vi "CVT2ReferenceWriteTest.vi"() -> (3 "Unit Test Framework Results":T1)   [LabVIEW 2013, in "UnitTests.lvlib"]
uses:
  UnitTests.lvlib
  <vilib>/utf/common/utf_test_result_troll.ctl
  <vilib>/utf/common/utf_test_result.ctl
  <vilib>/utf/common/utf_test_result_failure.ctl
  <vilib>/utf/common/utf_test_comparison_operators.ctl
  <vilib>/utf/common/utf_vi_tag.ctl
  <vilib>/NI/Current Value Table/Type Defs/Data Types.ctl
  <vilib>/NI/Current Value Table/DataTypes/I32_Write Index Set.vi
  <vilib>/NI/Current Value Table/DataTypes/I32_Read Index Set.vi
  <vilib>/NI/Current Value Table/FGVs/Tag Memory.vi
  <vilib>/NI/Current Value Table/Memory Block.vi
  <vilib>/NI/Current Value Table/DataTypes/I32_Memory Block.vi
  <vilib>/utf/NI_UnitTestFramework.lvlib
  <vilib>/NI/Current Value Table/Current Value Table.lvlib
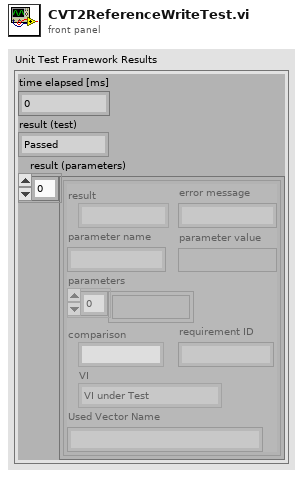
[diagram p1: front panel]
types:
  T1 = typedef "NI_UnitTestFramework.lvlib/utf_test_result_troll.ctl" = cluster{"time elapsed [ms]":u32, "result (test)":T2, "result (parameters)":T3[]}
  T2 = typedef "NI_UnitTestFramework.lvlib/utf_test_result.ctl" = enum16{"Passed", "Failed", "Error", "Skipped", "Not Processed"}
  T3 = typedef "NI_UnitTestFramework.lvlib/utf_test_result_failure.ctl" = cluster{"result":T2, "error message":string, "parameter name":string, "parameter value":variant, "parameters":variant[], "comparison":T4, "requirement ID":string, "VI":T5, "Used Vector Name":string}
  T4 = typedef "NI_UnitTestFramework.lvlib/utf_test_comparison_operators.ctl" = enum16{"=", "!=", ">", ">=", "<", "<=", "range", "symmetric tolerance", "asymmetric tolerance", "string contains", "string not contain", "array size", "string length", "array range", "by element", "array range (limit array)", "user-defined", "array contains", "array not contain", "vector length", "= (elm)", "!= (elm)", "= (case insensitive)", "!= (case insensitive)"}
  T5 = typedef "NI_UnitTestFramework.lvlib/utf_vi_tag.ctl" = enum16{"Setup VI", "VI under Test", "Teardown VI"}
  T6 = typedef "Current Value Table.lvlib/Data Types.ctl" = enum16{"Double", "Single", "I64", "I32", "I16", "I8", "U64", "U32", "U16", "U8", "String", "Boolean", "Array of U8", "Array of U16", "Array of U32", "Array of U64", "Array of I64", "Array of I32", "Array of I16", "Array of I8", "Array of Double", "Array of Single", "Array of Boolean", "Array of String"}
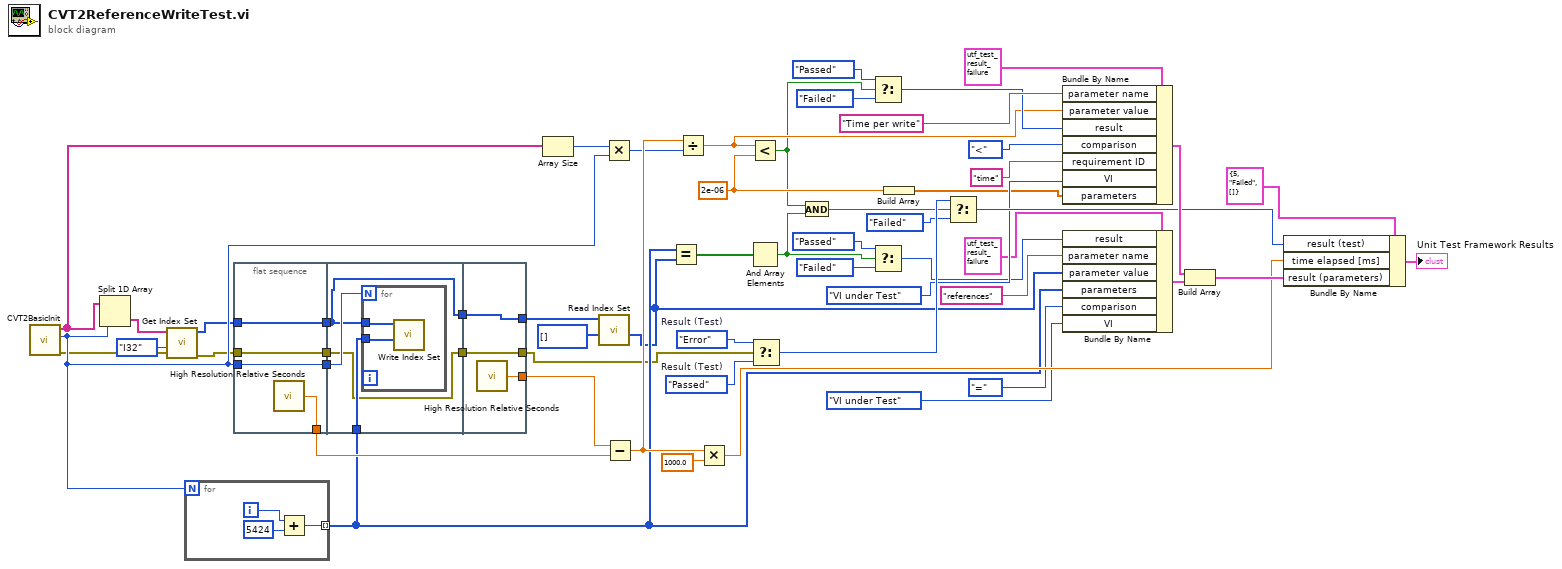
[diagram p0: block diagram]
diagram:
  w31 = 2e-06 ("y")
  w51 = utf_test_result."Error"  # Result (Test)
  w50 = utf_test_result."Passed"  # Result (Test)
  n1 = call "CVT2BasicInit.vi"() -> ("error out"=w12:errorcluster, "Tags per type out"=w13:i32, "names"=w14:string[])  [unwired: 9 in]
  n2 = Split 1D Array(array=w14, index=w13) -> (second subarray=w2:string[])  [unwired: 1 out]
  n3 = call <vilib>:"Get Index Set.vi"("error in (no error)"=w12, "Expected Type"=Data_Types."I32", "Tag Names"=w2) -> ("error out"=w11:errorcluster, "Tag References"=w9:i32[])  [unwired: 7 in]
  n4 = for {
    N: w13 -> [_]
    tunnel: [w57] -> w15 mode=indexing
    i -> [w59]
    n5 = Add(x=w59, y=5424) -> (x+y=w57:i32)
  }
  n6 = flat-sequence {
    tunnel: [w63] -> w53
    tunnel: w11 -> [w61]
    tunnel: [w62] -> w45
    tunnel: w13 -> [w62]
    tunnel: [w61] -> w44
    tunnel: w9 -> [w60]
    tunnel: [w60] -> w8
    tunnel: w45 -> [w67]
    tunnel: w44 -> [w65]
    tunnel: w15 -> [w66]
    tunnel: [w65] -> w10
    tunnel: w8 -> [w64]
    tunnel: [w64] -> w4
    tunnel: [w72] -> w54
    tunnel: [w71] -> w7
    tunnel: w10 -> [w71]
    tunnel: w4 -> [w70]
    tunnel: [w70] -> w3
    frame #0 {
      n7 = call <vilib>:"High Resolution Relative Seconds.vi"() -> ("relative seconds"=w63:dbl)
    }
    frame #1 {
      n8 = for {
        N: w67 -> [_]
        tunnel: w66 -> [w69]
        tunnel: w64 -> [w68]
        n9 = call-poly <vilib>:"Write Index Set.vi"("Values"=w69, "Indices"=w68) -> ()  [unwired: 10 in]
      }
    }
    frame #2 {
      n10 = call <vilib>:"High Resolution Relative Seconds.vi"() -> ("relative seconds"=w72:dbl)
    }
  }
  n11 = Array Size(array=w14) -> (size(s)=w26:i32)
  n12 = call-poly <vilib>:"Read Index Set.vi"("Default"=i32[] [], "Indices"=w3) -> ("Values"=w5:i32[])  [unwired: 9 in]
  n13 = Multiply(x=w26, y=w13) -> (x*y=w25:i32)
  n14 = Subtract(x=w54, y=w53) -> (x-y=w43:dbl)
  n15 = Equal?(x=w15, y=w5) -> (x = y?=w17:bool[])
  n16 = Divide(x=w43, y=w25) -> (x/y=w34:dbl)
  n17 = Multiply(x=w43, y=1000.0) -> (x*y=w46:dbl)
  n18 = Less?(x=w34, y=w31) -> (x < y?=w27:bool)
  n19 = And Array Elements(Boolean array=w17) -> (logical AND=w16:bool)
  n20 = Select(t=w51, s=w7, f=w50) -> (s? t:f=w41:T2)
  n21 = And(x=w27, y=w16) -> (x .and. y?=w28:bool)
  n22 = Select(t=utf_test_result."Passed" ("result"), s=w27, f=utf_test_result."Failed" ("result")) -> (s? t:f=w35:T2)
  n23 = Select(t=utf_test_result."Passed" ("result"), s=w16, f=utf_test_result."Failed" ("result")) -> (s? t:f=w20:T2)
  n24 = Build Array(w31) -> (w30:dbl[])
  n25 = Select(t=w41, s=w28, f=utf_test_result."Failed") -> (s? t:f=w39:T2)
  n26 = Bundle By Name(cluster=T3 {"result"=enum."Passed", "error message"="", "parameter name"="", "parameter value"=variant, "parameters"=[], "comparison"=enum."=", "requirement ID"="", "VI"=enum."Setup VI", "Used Vector Name"=""} ("Unit Test Framework - result (parameters)"), "parameter name"="Time per write", "parameter value"=w34, "result"=w35, "comparison"=utf_test_comparison_operators."<", "requirement ID"="time", "VI"=utf_vi_tag."VI under Test", "parameters"=w30) -> (w49:T3)
  n27 = Bundle By Name(cluster=T3 {"result"=enum."Passed", "error message"="", "parameter name"="", "parameter value"=variant, "parameters"=[], "comparison"=enum."=", "requirement ID"="", "VI"=enum."Setup VI", "Used Vector Name"=""} ("Unit Test Framework - result (parameters)"), "result"=w20, "parameter name"="references" ("format string"), "parameter value"=w5, "parameters"=w15, "comparison"=utf_test_comparison_operators."=", "VI"=utf_vi_tag."VI under Test") -> (w29:T3)
  n28 = Build Array(w49, w29) -> (w48:T3[])
  n29 = Bundle By Name(cluster=T1 {"time elapsed [ms]"=5, "result (test)"=enum."Failed", "result (parameters)"=[]} ("Unit Test Framework - Result"), "result (test)"=w39, "time elapsed [ms]"=w46, "result (parameters)"=w48) -> (→"Unit Test Framework Results":T1)
